vi "Remove Tag.vi"(8 "error in (no error)":errorcluster, 11 "FeedItem in":refnum<class "FeedItem.lvclass">) -> (0 "error out":errorcluster, 3 "FeedItem out":refnum<class "FeedItem.lvclass">)   [LabVIEW 2017, in "FeedItem.lvclass"]
uses:
  <vilib>/NI_RSS/FeedItem/FeedItem.lvclass
  <vilib>/NI_RSS/FeedItem/FeedItem.lvclass/FeedItem.ctl
panel:
  in  "Tag":string
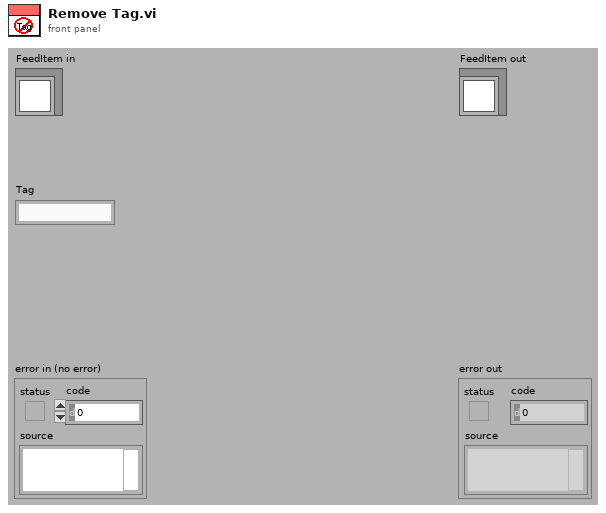
[diagram p1: front panel]
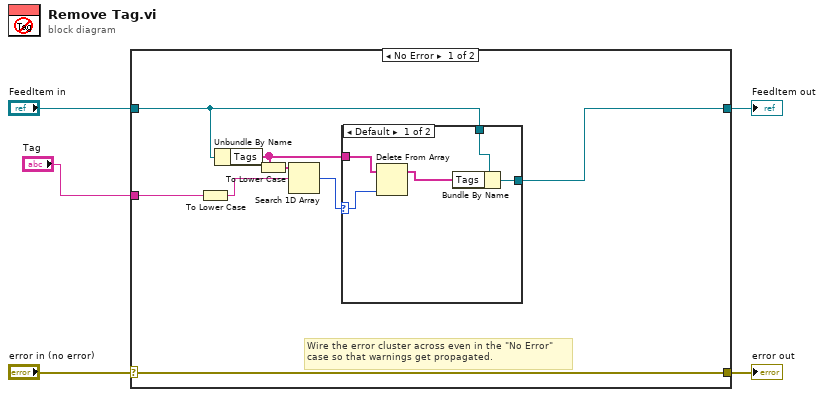
[diagram p0: block diagram]
diagram:
  n1 = case shown="No Error" "error in (no error)" {
    selector: "error in (no error)" -> [w13 w21]
    tunnel: [w13 w21] -> w4
    tunnel: [w6 w20] -> w2
    tunnel: "FeedItem in" -> [w7 w20]
    tunnel: "Tag" -> [w11 _]
    frame No Error {
      # "Wire the error cluster across even in the \"No Error\"\ncase so that warnings get propagated."
      n2 = To Lower Case(string=w11) -> (all lower case string=w10:string)
      n3 = Unbundle By Name(w7) -> ("Tags"=w8:string[])
      n4 = To Lower Case(string=w8) -> (all lower case string=w12:string[])
      n5 = Search 1D Array(1D array=w12, element=w10) -> (index of element=w9:i32)  [unwired: 1 out]
      n6 = case shown="Default" w9 {
        selector: w9 -> [w16 _]
        tunnel: w7 -> [w18 w19]
        tunnel: w8 -> [w17 _]
        tunnel: [w14 w19] -> w6
        frame Default {
          n7 = Delete From Array(array=w17, index=w16) -> (array with subset deleted=w15:string[])  [unwired: 1 in, 1 out]
          n8 = Bundle By Name(cluster=w18, "Tags"=w15) -> (w14:refnum<class "FeedItem.lvclass">)
        }
        frame -1 {
        }
      }
    }
    frame Error {
    }
  }
  "error out" <- w4
  "FeedItem out" <- w2
